vi "Read Serial data array.vi"(8 "error in (no error)":errorcluster, 11 "Serial Array in":refnum<visa-resource-name>[](array[refnum])) -> (0 "error out":errorcluster, 1 "Serial cluster array":T1[](array[typedef]), 2 "Buffer array":string[](array[string]), 3 "Serial Array out":refnum<visa-resource-name>[](array[refnum]), 5 "Trip pressure array":dbl[](array[numeric]))   [LabVIEW 2019]
uses:
  Labview clones/AML-UHV-Gauge-Controller/lvsrc/sandbox/Instrument.AML.GetAll--Cluster.ctl
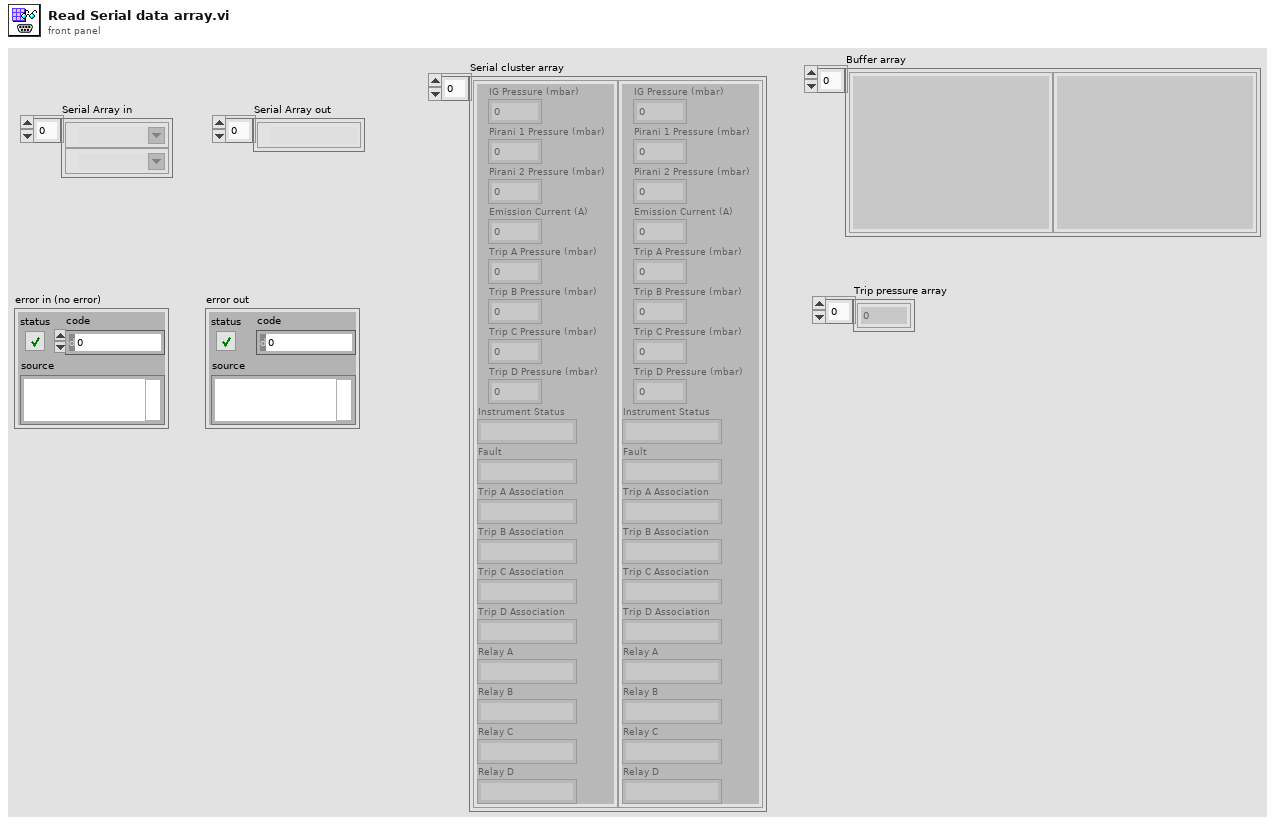
[diagram p1: front panel]
types:
  T1 = typedef "Instrument.AML.GetAll--Cluster.ctl" = cluster{"IG Pressure (mbar)":dbl, "Pirani 1 Pressure (mbar)":dbl, "Pirani 2 Pressure (mbar)":dbl, "Emission Current (A)":dbl, "Trip A Pressure (mbar)":dbl, "Trip B Pressure (mbar)":dbl, "Trip C Pressure (mbar)":dbl, "Trip D Pressure (mbar)":dbl, "Instrument Status":string, "Fault":string, "Trip A Association":string, "Trip B Association":string, "Trip C Association":string, "Trip D Association":string, "Relay A":string, "Relay B":string, "Relay C":string, "Relay D":string}
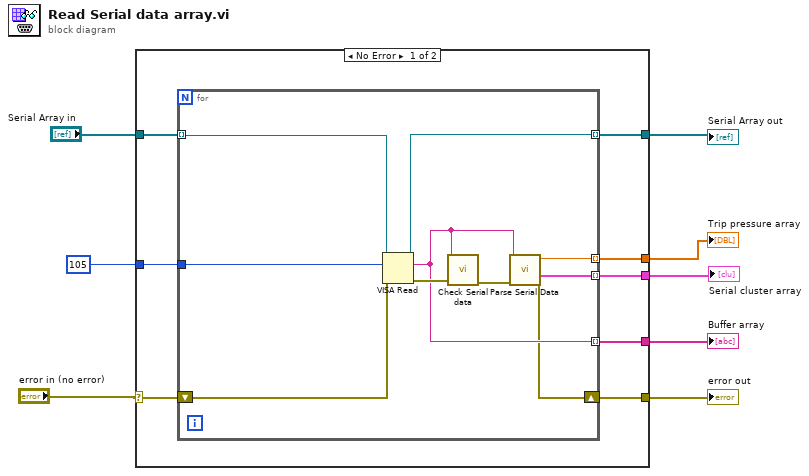
[diagram p0: block diagram]
diagram:
  n1 = case shown="No Error" "error in (no error)" {
    selector: "error in (no error)" -> [w14 w28]
    tunnel: u32 105 ("byte count") -> [w16 _]
    tunnel: [w15 w28] -> w7
    tunnel: [w13 w27] -> w5
    tunnel: "Serial Array in" -> [w12 w27]
    tunnel: [w11 _] -> w3
    tunnel: [w10 _] -> w2
    tunnel: [w9 _] -> w1
    frame No Error {
      n2 = for {
        tunnel: [w20] -> w11 mode=indexing
        tunnel: w16 -> [w26]
        shift-right: [w19] -> w15
        shift-left: w14 -> [w25]
        tunnel: [w24] -> w13 mode=indexing
        tunnel: w12 -> [w23] mode=indexing
        tunnel: [w18] -> w10 mode=indexing
        tunnel: [w17] -> w9 mode=indexing
        n3 = VISA Read(VISA resource name=w23, byte count=w26, error in (no error)=w25) -> (VISA resource name out=w24:refnum<visa-resource-name>, read buffer=w20:string, error out=w22:errorcluster)  [unwired: 1 out]
        n4 = call "Check Serial data.vi"("error in"=w22, "Buffer in"=w20) -> ("error IO"=w21:errorcluster)  [unwired: 8 in, 1 out]
        n5 = call "Parse Serial Data.vi"("error in"=w21, "Buffer in"=w20) -> ("error IO"=w19:errorcluster, "cluster"=w18:T1, "Trip pressure"=w17:dbl)  [unwired: 7 in]
      }
    }
    frame Error {
    }
  }
  "error out" <- w7
  "Serial Array out" <- w5
  "Serial cluster array" <- w2
  "Buffer array" <- w3
  "Trip pressure array" <- w1
